vi "ConfigureSounds.vi"(11 "File":string="soundconfig.xml") -> (1 "Sound Cluster":T1={"Start"={"total number of samples/ch"=31680, "sound format"={"sample rate (S/s)"=11025.0, "number of channels"=1, "bits per sample"=16}, "data"=[{"t0"=timestamp(0 s since 1904-01-01), "dt"=9.070294784580499e-05, "Y"=array[31680 elements]}], "Volume"=100.0}, "Stop"={"total number of samples/ch"=27648, "sound format"={"sample rate (S/s)"=11025.0, "number of channels"=1, "bits per sample"=16}, "data"=[{"t0"=timestamp(0 s since 1904-01-01), "dt"=9.070294784580499e-05, "Y"=array[27648 elements]}], "Volume"=100.0}, "Uh-Oh"={"total number of samples/ch"=29952, "sound format"={"sample rate (S/s)"=11025.0, "number of channels"=1, "bits per sample"=16}, "data"=[{"t0"=timestamp(0 s since 1904-01-01), "dt"=9.070294784580499e-05, "Y"=array[29952 elements]}], "Volume"=88.46153846153847}, "PreMatch"={"total number of samples/ch"=225792, "sound format"={"sample rate (S/s)"=44100.0, "number of channels"=2, "bits per sample"=16}, "data"=[{"t0"=timestamp(0 s since 1904-01-01), "dt"=2.2675736961451248e-05, "Y"=array[225792 elements]}, {"t0"=timestamp(0 s since 1904-01-01), "dt"=2.2675736961451248e-05, "Y"=array[225792 elements]}], "Volume"=75.38461538461539}, "Hurry-Up"={"total number of samples/ch"=0, "sound format"={"sample rate (S/s)"=0.0, "number of channels"=0, "bits per sample"=0}, "data"=[], "Volume"=0.0}}, 3 "output cluster":T4)   [LabVIEW 2013]
uses:
  Sound Info.ctl
  <vilib>/sound2/lvsound2.llb/Sound Data Format.ctl
  <vilib>/Utility/sysdir.llb/System Directory Type.ctl
  <vilib>/sound2/lvsound2.llb/Sampling Mode.ctl
  <vilib>/Utility/xml.llb/Read From XML File(string).vi
  <vilib>/Utility/xml.llb/Write to XML File(string).vi
  <vilib>/sound2/lvsound2.llb/Sound Output Set Volume (Single).vi
  <vilib>/sound2/lvsound2.llb/Sound Output Write (DBL).vi
panel:
  in  "stop":bool
  in  "Sound To Play":T3(ring)
  in  "Tab Control":enum32{"Page 1", "Page 2"}(tab)
  in  "Cancel Button":bool
  in  "OK Button":bool
  in  "Test Hurry Up Sound":bool
  in  "Load Hurry Up Sound":bool
  in  "Hurry Up Sound Volume":dbl(slide)=88.46153846153847 scale=0.0..100.0
  in  "Hurry Up Sound":path=path "C:/ProgramData/FLL/sounds/TimeToRun.wav"
  in  "Test Pre-Match Sound":bool
  in  "Load Pre-Match Sound":bool
  in  "Pre-Match Coundown Sound Volume":dbl(slide)=88.46153846153847 scale=0.0..100.0
  in  "Pre-Match Countdown Sound":path=path "Z:/Code/LabVIEW/FLL 2.1/sounds/FOGHORN.wav"
  in  "Test Uh-Oh Sound":bool
  in  "Load Uh-Oh Sound":bool
  in  "Uh-Oh Sound Volume":dbl(slide)=88.46153846153847 scale=0.0..100.0
  in  "Uh-Oh Sound Path":path=path "Z:/Code/LabVIEW/FLL 2.1/sounds/FOGHORN.wav"
  in  "Test Stop Sound":bool
  in  "Load Stop Sound":bool
  in  "Stop Sound Volume":dbl(slide)=100.0 scale=0.0..100.0
  in  "Stop Sound Path":path=path "Z:/Code/LabVIEW/FLL 2.1/sounds/BUZZER.wav"
  in  "Test Start Sound":bool
  in  "Load Start Sound":bool
  in  "Start Sound Volume":dbl(slide)=100.0 scale=0.0..100.0
  in  "Start Sound Path":path=path "Z:/Code/LabVIEW/FLL 2.1/sounds/CHARGE.wav"
  in  "Master Volume":dbl(slide)=100.0 min=1.0 scale=0.0..100.0
  in  "Secondary (s)":dbl
  in  "Primary (s)":dbl=150.0
  in  "Pre-Primary (s)":dbl
  # "5"
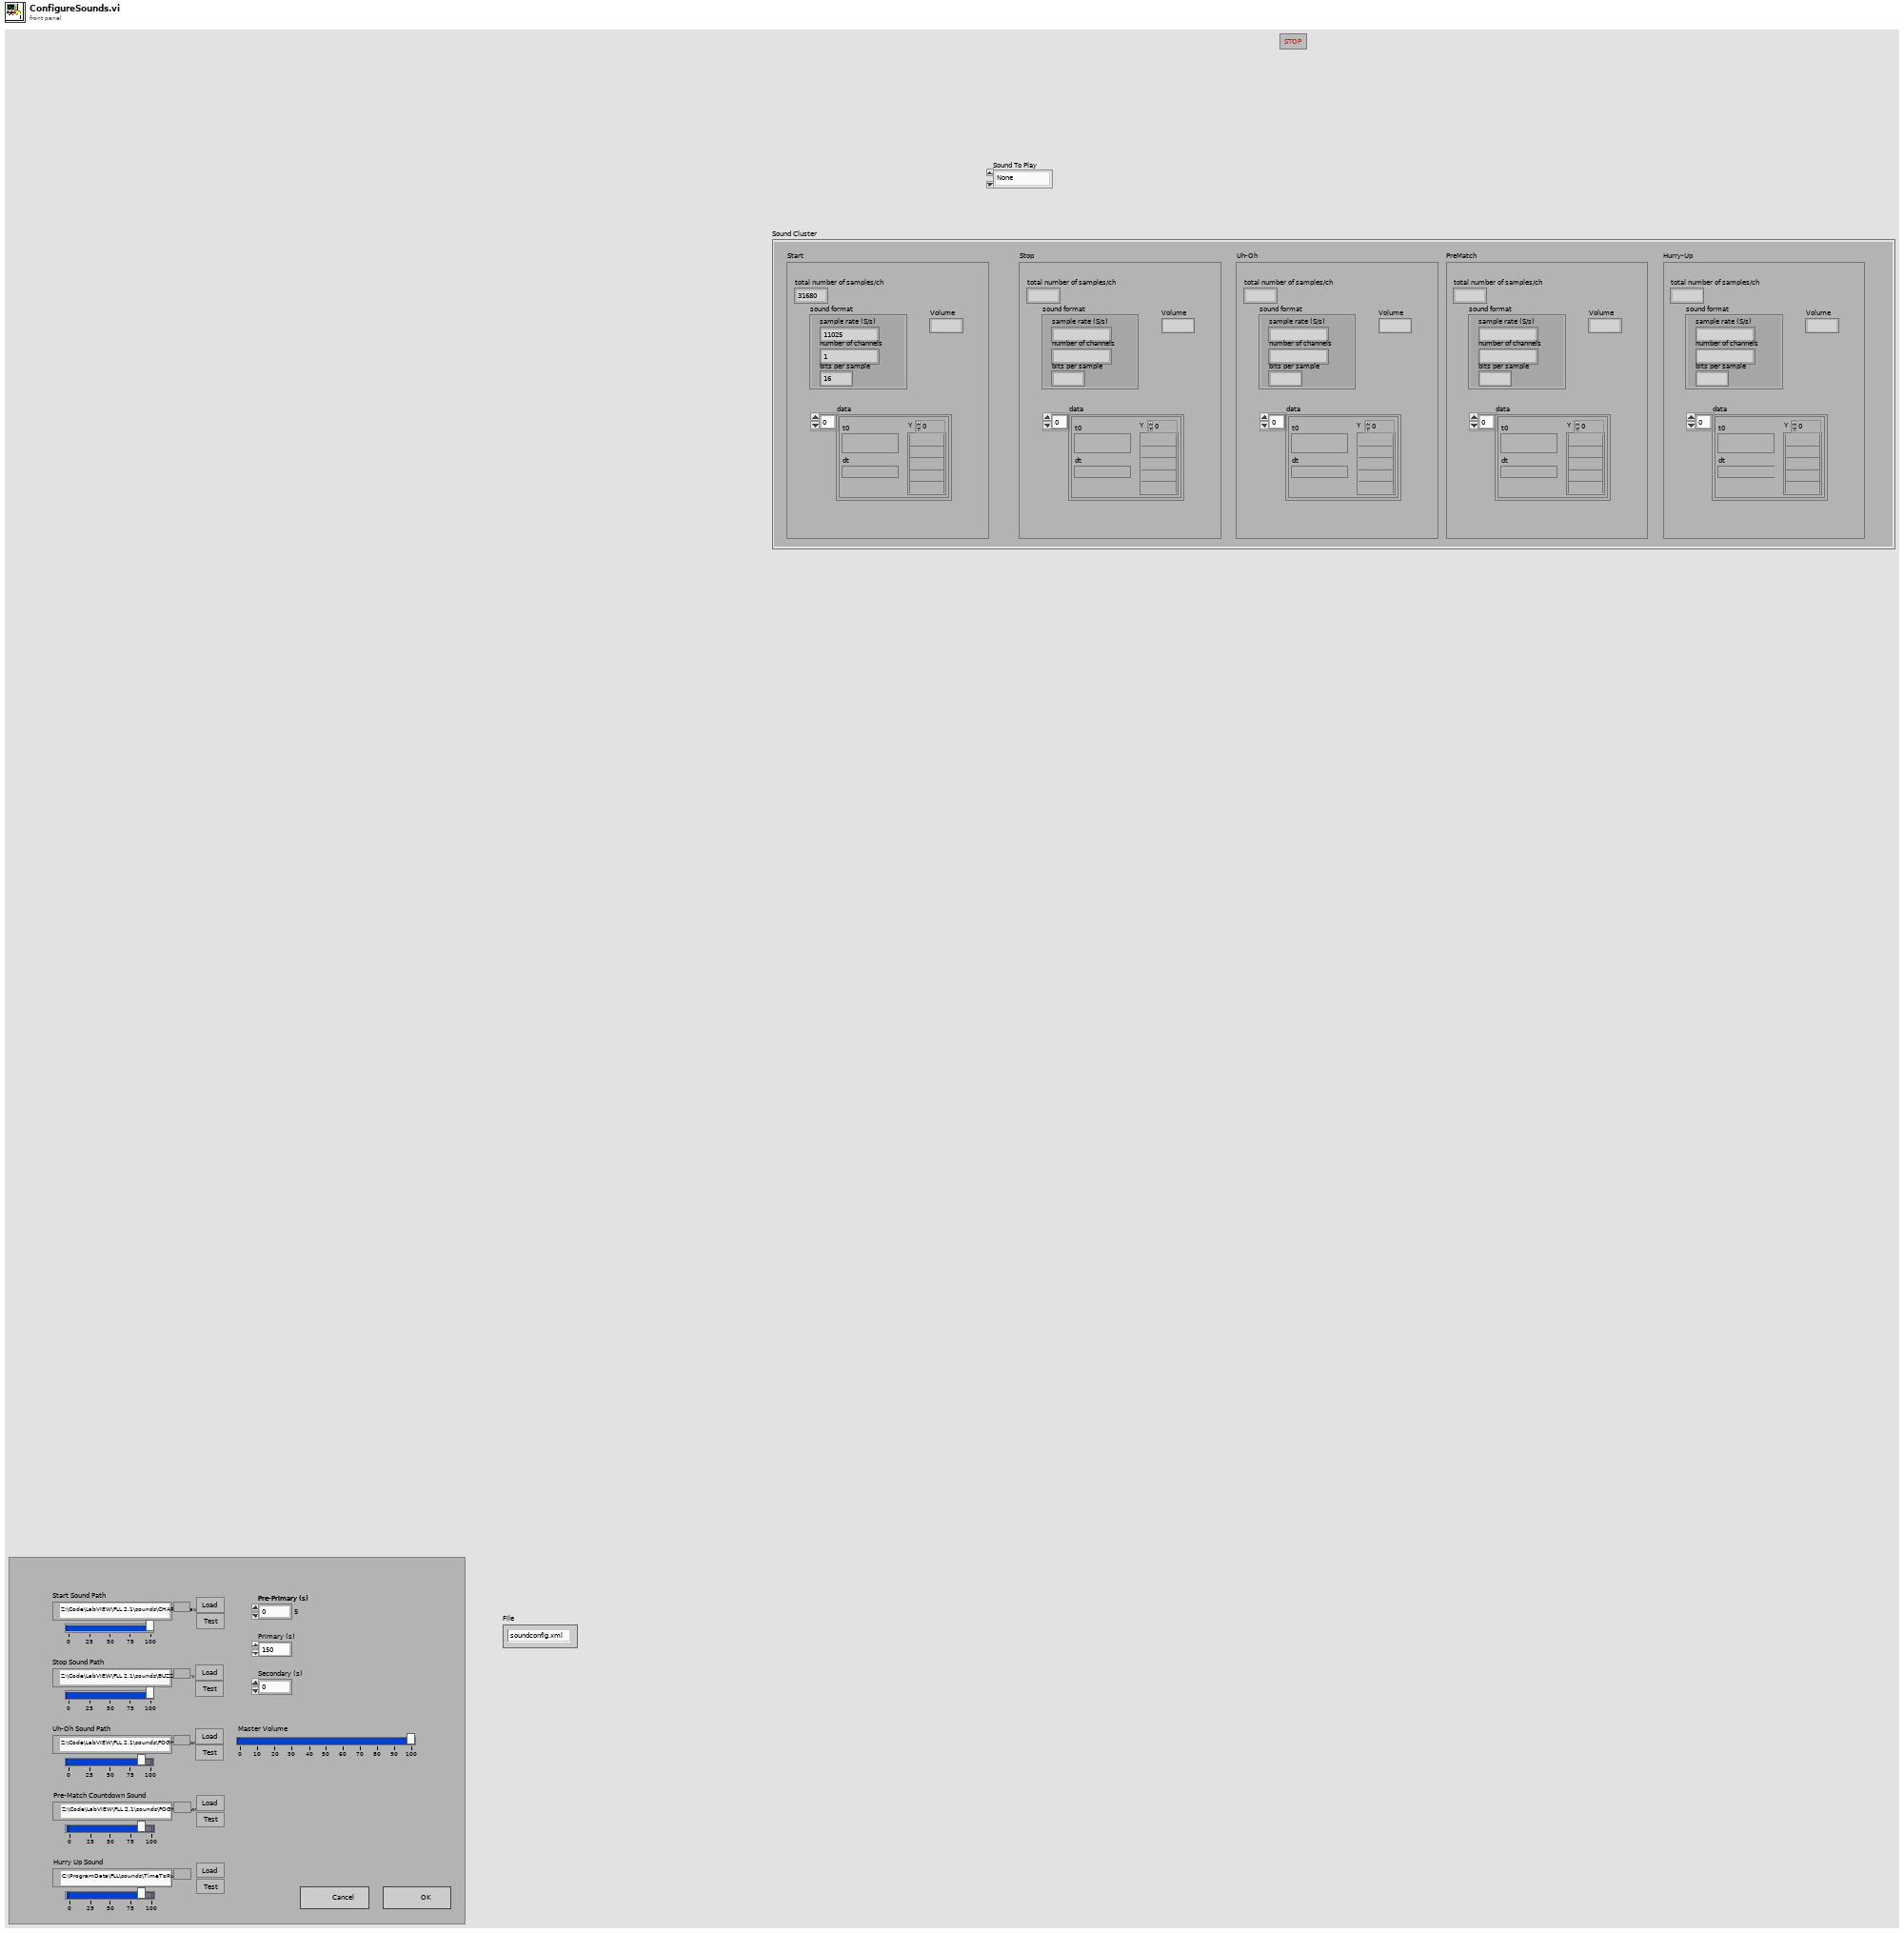
[diagram p1: front panel]
types:
  T1 = typedef "Sound Info.ctl" = cluster{"Start":cluster{"total number of samples/ch":u32, "sound format":T2, "data":waveform(dbl)[], "Volume":dbl}, "Stop":cluster{"total number of samples/ch":u32, "sound format":T2, "data":waveform(dbl)[], "Volume":dbl}, "Uh-Oh":cluster{"total number of samples/ch":u32, "sound format":T2, "data":waveform(dbl)[], "Volume":dbl}, "PreMatch":cluster{"total number of samples/ch":u32, "sound format":T2, "data":waveform(dbl)[], "Volume":dbl}, "Hurry-Up":cluster{"total number of samples/ch":u32, "sound format":T2, "data":waveform(dbl)[], "Volume":dbl}}
  T2 = typedef "Sound Data Format.ctl" = cluster{"sample rate (S/s)":dbl, "number of channels":i32, "bits per sample":i32}
  T3 = enum16{"None", "Start", "Stop", "Uh-Oh", "Prematch", "Hurry-Up"}
  T4 = cluster{"Master Volume":dbl, "Pre-Primary (s)":dbl, "Primary (s)":dbl, "Secondary (s)":dbl, "Start Sound Path":path, "Stop Sound Path":path, "Uh-Oh Sound Path":path, "Pre-Match Countdown Sound":path, "Hurry Up Sound":path, "Start Sound Volume":dbl, "Stop Sound Volume":dbl, "Uh-Oh Sound Volume":dbl, "Pre-Match Coundown Sound Volume":dbl, "Hurry Up Sound Volume":dbl}
  T5 = typedef "System Directory Type.ctl" = i32
  T6 = cluster{"total number of samples/ch":u32, "sound format":T2, "data":waveform(dbl)[], "Volume":dbl}
  T7 = typedef "Sampling Mode.ctl" = i32
  T8 = typedef "Sound Output Task ID.ctl" = u32
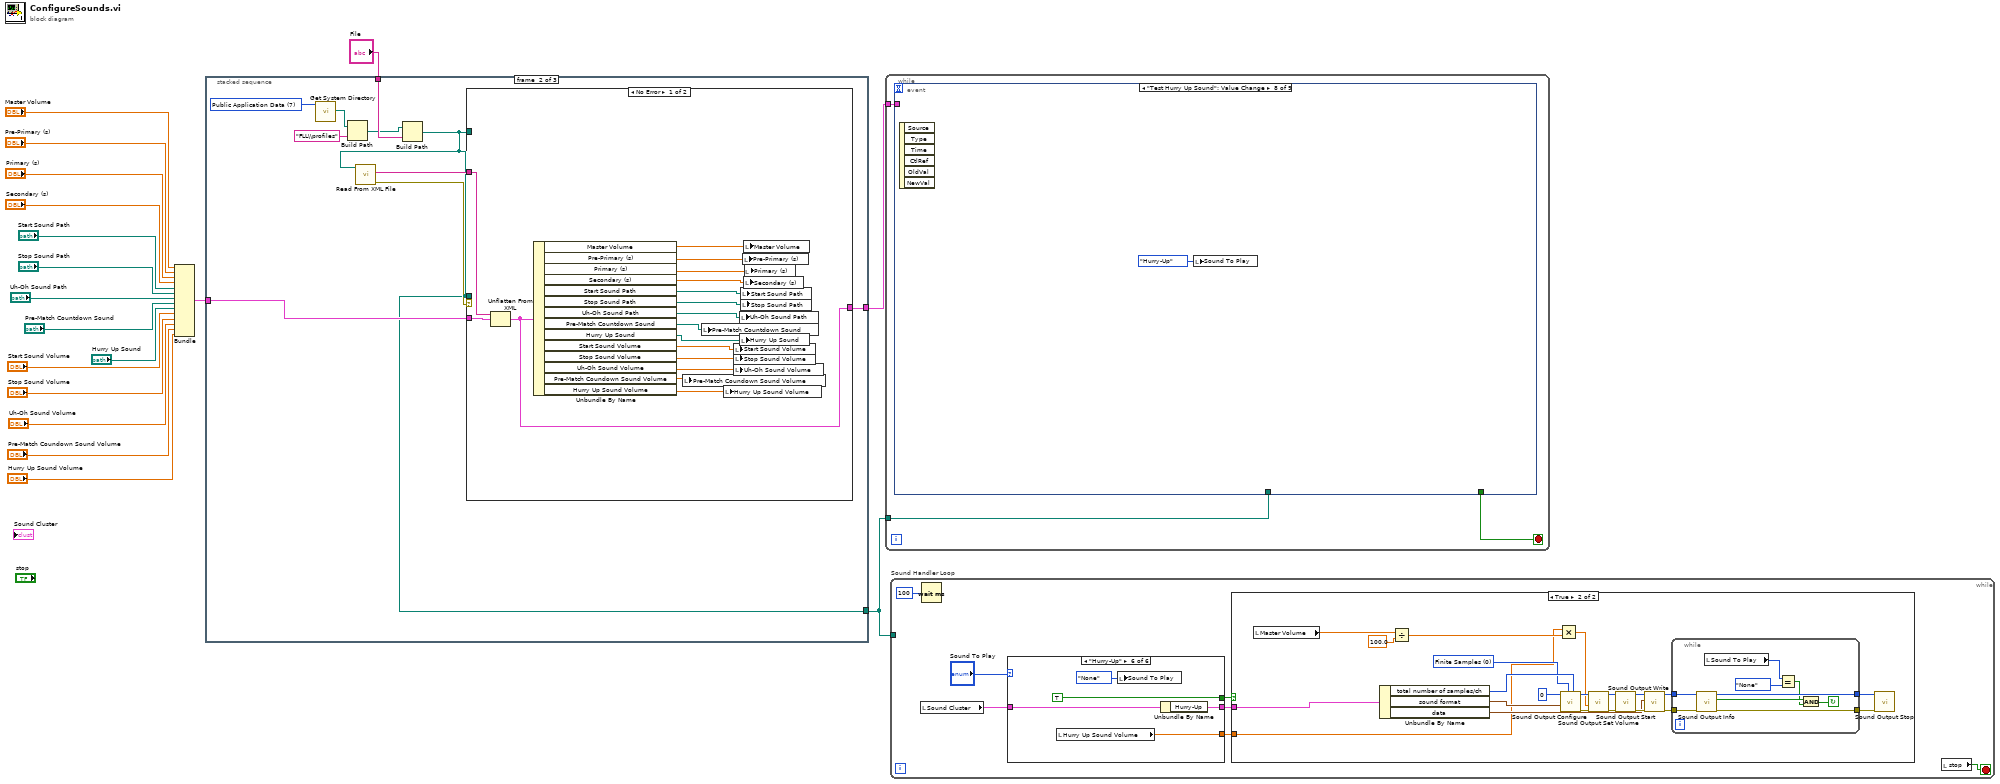
[diagram p0: block diagram]
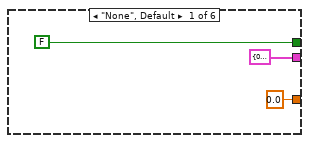
[diagram p3: hidden frame]
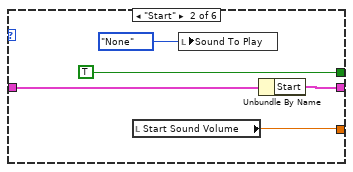
[diagram p4: hidden frame]
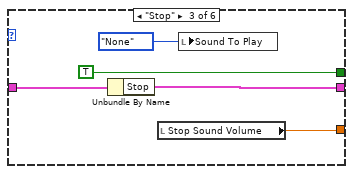
[diagram p5: hidden frame]
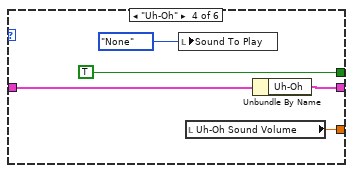
[diagram p6: hidden frame]
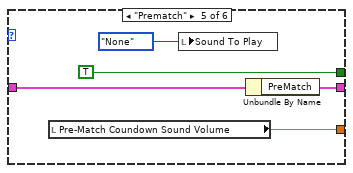
[diagram p7: hidden frame]
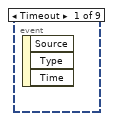
[diagram p8: hidden frame]
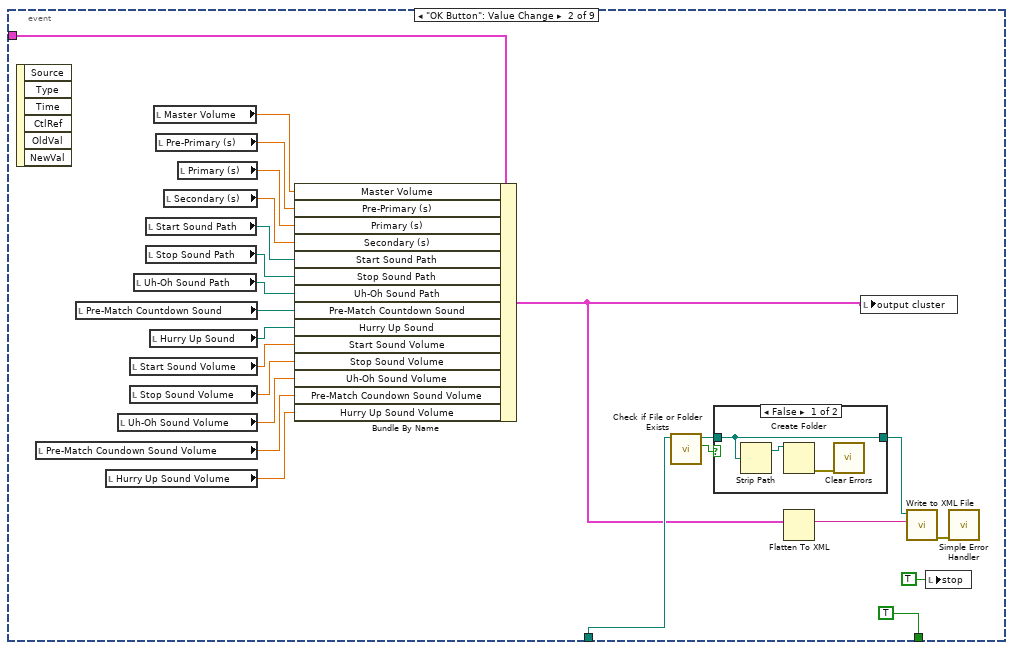
[diagram p9: hidden frame]
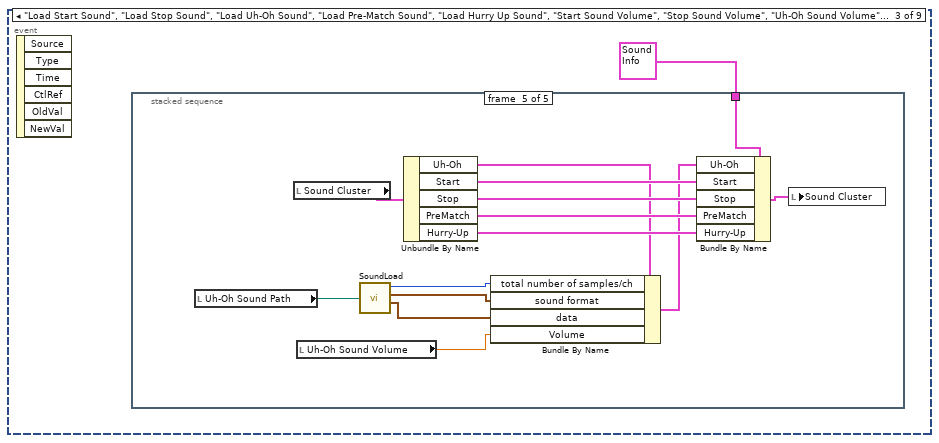
[diagram p11: hidden frame]
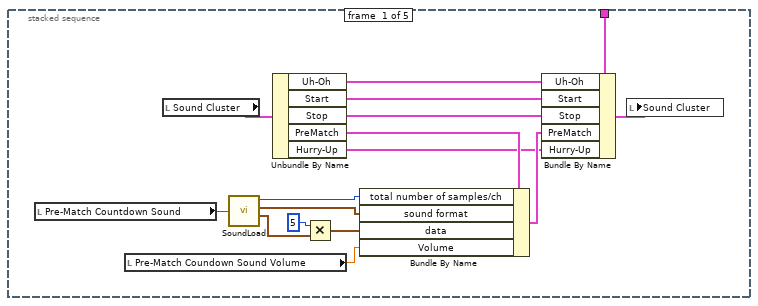
[diagram p12: hidden frame]
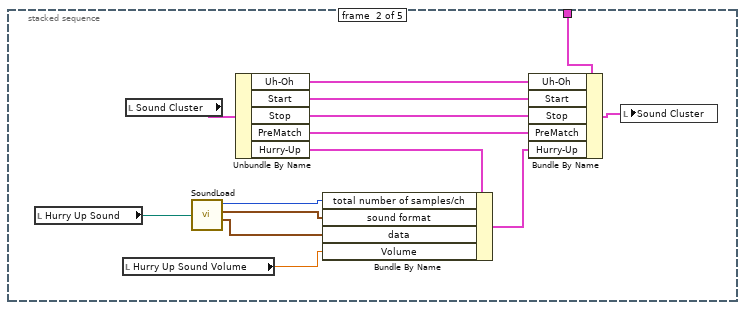
[diagram p13: hidden frame]
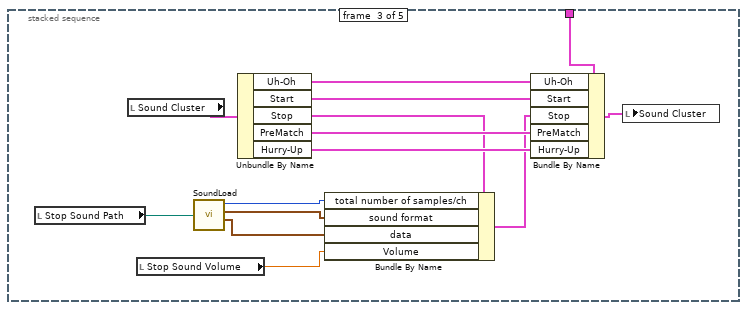
[diagram p14: hidden frame]
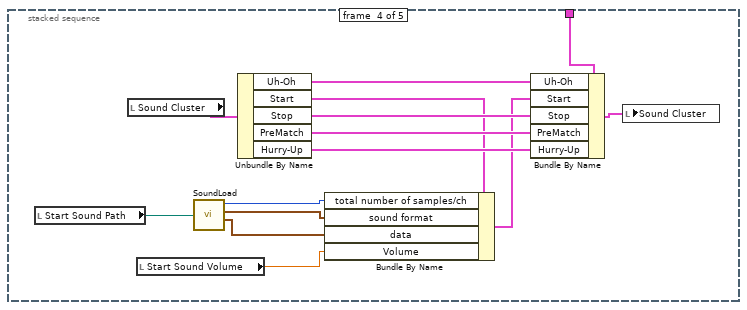
[diagram p15: hidden frame]
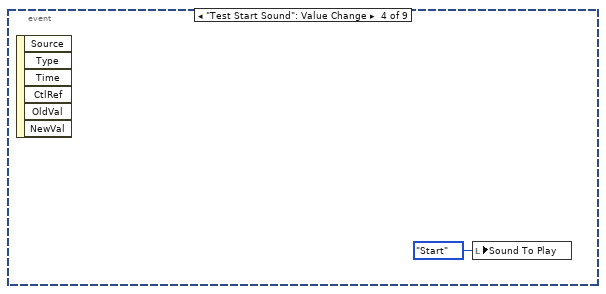
[diagram p16: hidden frame]
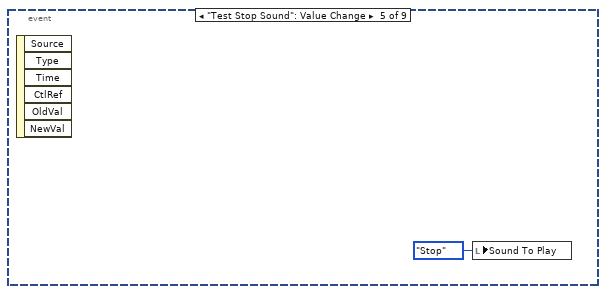
[diagram p17: hidden frame]
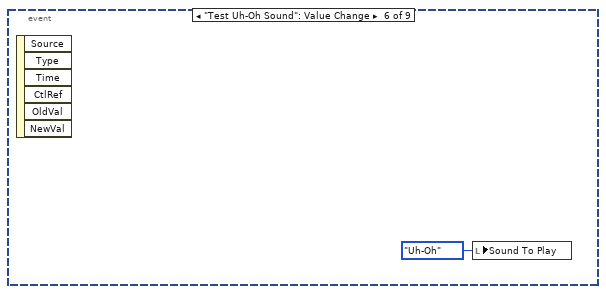
[diagram p18: hidden frame]
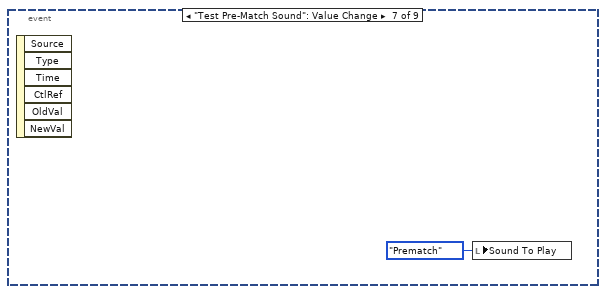
[diagram p19: hidden frame]
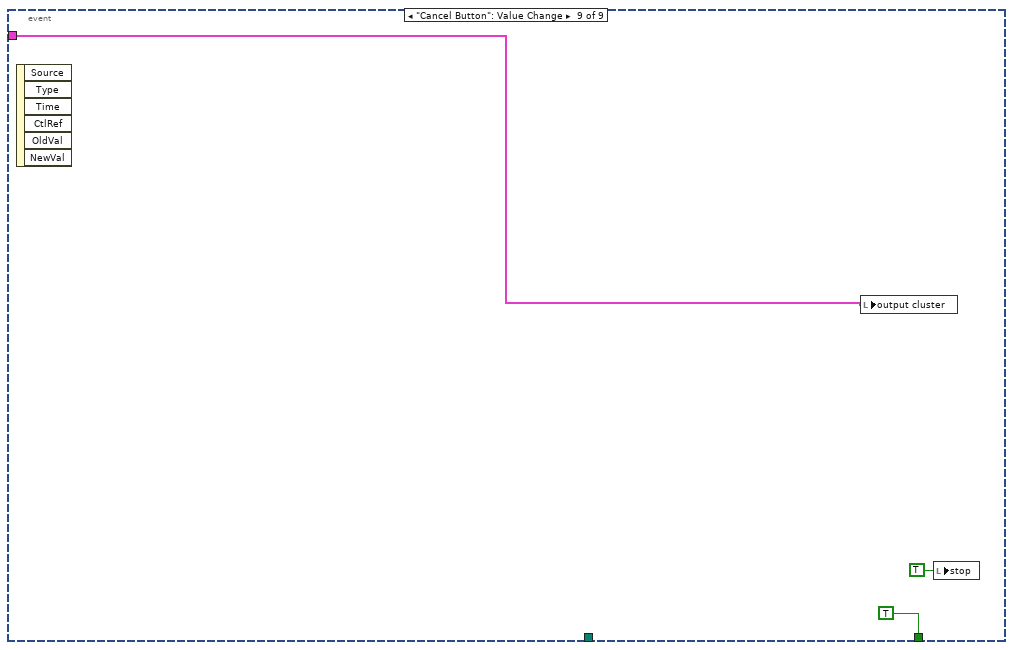
[diagram p20: hidden frame]
diagram:
  n1 = Bundle("Master Volume"="Master Volume", "Pre-Primary (s)"="Pre-Primary (s)", "Primary (s)"="Primary (s)", "Secondary (s)"="Secondary (s)", "Start Sound Path"="Start Sound Path", "Stop Sound Path"="Stop Sound Path", "Uh-Oh Sound Path"="Uh-Oh Sound Path", "Pre-Match Countdown Sound"="Pre-Match Countdown Sound", "Hurry Up Sound"="Hurry Up Sound", "Start Sound Volume"="Start Sound Volume", "Stop Sound Volume"="Stop Sound Volume", "Uh-Oh Sound Volume"="Uh-Oh Sound Volume", "Pre-Match Coundown Sound Volume"="Pre-Match Coundown Sound Volume", "Hurry Up Sound Volume"="Hurry Up Sound Volume") -> (w4:T4)  [unwired: 1 in]
  n2 = stacked-sequence {
    tunnel: w4 -> [_ w36 _]
    tunnel: [_ w31 _] -> w2
    tunnel: [_ w34 _] -> w3
    tunnel: "File" -> [_ w33 _]
    frame #0 {
      n3 = local write "stop"(FALSE ("stop")) -> ()
      n4 = control-ref of="Test Pre-Match Sound"() -> (w25:refnum<vi>)
      n5 = control-ref of="Test Hurry Up Sound"() -> (w26:refnum<vi>)
      n6 = control-ref of="Test Uh-Oh Sound"() -> (w24:refnum<vi>)
      n7 = control-ref of="Test Stop Sound"() -> (w23:refnum<vi>)
      n8 = control-ref of="Test Start Sound"() -> (w22:refnum<vi>)
      n9 = control-ref of="Cancel Button"() -> (w28:refnum<vi>)
      n10 = control-ref of="OK Button"() -> (w27:refnum<vi>)
      n11 = Build Array(w28, w27, w26, w25, w24, w23, w22) -> (w21:refnum<vi>[])
      n12 = for {
        tunnel: w21 -> [w30] mode=indexing
        n13 = property class="Bool (strict)"(reference=w30, "Value"=FALSE) -> ()  [unwired: 1 in, 2 out]
      }
      n14 = local write "Tab Control"(enum32{"Page 1", "Page 2"}."Page 1" ("Tab Control")) -> ()
    }
    frame #1 {
      w40 = T5 7 items=["User Home"=0, "User Desktop"=1, "User Documents"=2, "User Application Data"=3, "User Preferences"=4, "User Temporary"=5, "Public Documents"=6, "Public Application Data"=7, "Public Preferences"=8, "Public Cache"=13, "System Core Libraries"=9, "System Installed Libraries"=10, "Application Files"=11, "Boot Volume Root"=12] ("system directory type")
      n15 = call <vilib>:"Get System Directory.vi"("system directory type"=w40) -> ("system directory"=w39:path)  [unwired: 10 in]
      n16 = Build Path(base path=w39, name or relative path="FLL\\profiles") -> (appended path=w32:path)
      n17 = Build Path(base path=w32, name or relative path=w33) -> (appended path=w31:path)
      n18 = call-poly <vilib>:"Read From XML File.vi"("XML File Path"=w31) -> ("error out"=w37:errorcluster, "XML Elements"=w35:string)  [unwired: 8 in, 1 out]
      n19 = case shown="No Error" w37 {
        tunnel: w31 -> [_ _]
        tunnel: w36 -> [w57 w58]
        tunnel: w35 -> [w56 _]
        tunnel: w31 -> [_ w61]
        tunnel: [w41 w58] -> w34
        frame No Error {
          n20 = Unflatten From XML(xml string=w56, type=w57) -> (value=w41:T4)  [unwired: 1 in, 1 out]
          n21 = Unbundle By Name(w41) -> ("Master Volume"=w55:dbl, "Pre-Primary (s)"=w54:dbl, "Primary (s)"=w53:dbl, "Secondary (s)"=w52:dbl, "Start Sound Path"=w51:path, "Stop Sound Path"=w50:path, "Uh-Oh Sound Path"=w49:path, "Pre-Match Countdown Sound"=w48:path, "Hurry Up Sound"=w47:path, "Start Sound Volume"=w46:dbl, "Stop Sound Volume"=w45:dbl, "Uh-Oh Sound Volume"=w44:dbl, "Pre-Match Coundown Sound Volume"=w43:dbl, "Hurry Up Sound Volume"=w42:dbl)
          n22 = local write "Pre-Match Coundown Sound Volume"(w43) -> ()
          n23 = local write "Pre-Match Countdown Sound"(w48) -> ()
          n24 = local write "Hurry Up Sound Volume"(w42) -> ()
          n25 = local write "Start Sound Volume"(w46) -> ()
          n26 = local write "Stop Sound Volume"(w45) -> ()
          n27 = local write "Uh-Oh Sound Volume"(w44) -> ()
          n28 = local write "Uh-Oh Sound Path"(w49) -> ()
          n29 = local write "Hurry Up Sound"(w47) -> ()
          n30 = local write "Start Sound Path"(w51) -> ()
          n31 = local write "Stop Sound Path"(w50) -> ()
          n32 = local write "Pre-Primary (s)"(w54) -> ()
          n33 = local write "Master Volume"(w55) -> ()
          n34 = local write "Secondary (s)"(w52) -> ()
          n35 = local write "Primary (s)"(w53) -> ()
        }
        frame Error {
          n36 = Path To String(path=w61) -> (string=w60:string)
          n37 = call "Build Text"("configfile"=w60) -> ("Result"=w59:string)  [unwired: 13 in, 1 out]
          n38 = call "Display Message to User"("Message"=w59) -> ()  [unwired: 9 in, 2 out]
        }
      }
    }
    frame #2 {
      n39 = stacked-sequence {
        tunnel: T1 {"Start"={"total number of samples/ch"=0, "sound format"={"sample rate (S/s)"=0.0, "number of channels"=0, "bits per sample"=0}, "data"=[], "Volume"=0.0}, "Stop"={"total number of samples/ch"=0, "sound format"={"sample rate (S/s)"=0.0, "number of channels"=0, "bits per sample"=0}, "data"=[], "Volume"=0.0}, "Uh-Oh"={"total number of samples/ch"=0, "sound format"={"sample rate (S/s)"=0.0, "number of channels"=0, "bits per sample"=0}, "data"=[], "Volume"=0.0}, "PreMatch"={"total number of samples/ch"=0, "sound format"={"sample rate (S/s)"=0.0, "number of channels"=0, "bits per sample"=0}, "data"=[], "Volume"=0.0}, "Hurry-Up"={"total number of samples/ch"=0, "sound format"={"sample rate (S/s)"=0.0, "number of channels"=0, "bits per sample"=0}, "data"=[], "Volume"=0.0}} ("Sound Info") -> [w77 w91 w105 w119 w133]
        frame #0 {
          n40 = local read "Pre-Match Countdown Sound"() -> (w68:path)
          n41 = local read "Pre-Match Coundown Sound Volume"() -> (w67:dbl)
          n42 = local read "Sound Cluster"() -> (w78:T1)
          n43 = call "SoundLoad.vi"("Sound File"=w68) -> ("total number of samples/ch"=w71:u32, "sound format"=w72:T2, "data"=w65:waveform(dbl)[])  [unwired: 1 out]
          n44 = Unbundle By Name(w78) -> ("Uh-Oh"=w69:T6, "Start"=w76:T6, "Stop"=w75:T6, "PreMatch"=w74:T6, "Hurry-Up"=w63:T6)
          n45 = Multiply(x=5, y=w65) -> (x*y=w64:waveform(dbl)[])
          n46 = Bundle By Name(cluster=w74, "total number of samples/ch"=w71, "sound format"=w72, "data"=w64, "Volume"=w67) -> (w73:T6)
          n47 = Bundle By Name(cluster=w77, "Uh-Oh"=w69, "Start"=w76, "Stop"=w75, "PreMatch"=w73, "Hurry-Up"=w63) -> (w70:T1)
          n48 = local write "Sound Cluster"(w70) -> ()
        }
        frame #1 {
          n49 = local read "Hurry Up Sound"() -> (w84:path)
          n50 = local read "Hurry Up Sound Volume"() -> (w83:dbl)
          n51 = local read "Sound Cluster"() -> (w92:T1)
          n52 = call "SoundLoad.vi"("Sound File"=w84) -> ("total number of samples/ch"=w87:u32, "sound format"=w88:T2, "data"=w79:waveform(dbl)[])  [unwired: 1 out]
          n53 = Unbundle By Name(w92) -> ("Uh-Oh"=w85:T6, "Start"=w90:T6, "Stop"=w89:T6, "PreMatch"=w82:T6, "Hurry-Up"=w81:T6)
          n54 = Bundle By Name(cluster=w81, "total number of samples/ch"=w87, "sound format"=w88, "data"=w79, "Volume"=w83) -> (w80:T6)
          n55 = Bundle By Name(cluster=w91, "Uh-Oh"=w85, "Start"=w90, "Stop"=w89, "PreMatch"=w82, "Hurry-Up"=w80) -> (w86:T1)
          n56 = local write "Sound Cluster"(w86) -> ()
        }
        frame #2 {
          n57 = local read "Stop Sound Path"() -> (w99:path)
          n58 = local read "Sound Cluster"() -> (w106:T1)
          n59 = local read "Stop Sound Volume"() -> (w98:dbl)
          n60 = call "SoundLoad.vi"("Sound File"=w99) -> ("total number of samples/ch"=w102:u32, "sound format"=w103:T2, "data"=w93:waveform(dbl)[])  [unwired: 1 out]
          n61 = Unbundle By Name(w106) -> ("Uh-Oh"=w100:T6, "Start"=w104:T6, "Stop"=w95:T6, "PreMatch"=w97:T6, "Hurry-Up"=w96:T6)
          n62 = Bundle By Name(cluster=w95, "total number of samples/ch"=w102, "sound format"=w103, "data"=w93, "Volume"=w98) -> (w94:T6)
          n63 = Bundle By Name(cluster=w105, "Uh-Oh"=w100, "Start"=w104, "Stop"=w94, "PreMatch"=w97, "Hurry-Up"=w96) -> (w101:T1)
          n64 = local write "Sound Cluster"(w101) -> ()
        }
        frame #3 {
          n65 = local read "Start Sound Path"() -> (w114:path)
          n66 = local read "Sound Cluster"() -> (w120:T1)
          n67 = local read "Start Sound Volume"() -> (w113:dbl)
          n68 = call "SoundLoad.vi"("Sound File"=w114) -> ("total number of samples/ch"=w117:u32, "sound format"=w118:T2, "data"=w107:waveform(dbl)[])  [unwired: 1 out]
          n69 = Unbundle By Name(w120) -> ("Uh-Oh"=w115:T6, "Start"=w109:T6, "Stop"=w110:T6, "PreMatch"=w112:T6, "Hurry-Up"=w111:T6)
          n70 = Bundle By Name(cluster=w109, "total number of samples/ch"=w117, "sound format"=w118, "data"=w107, "Volume"=w113) -> (w108:T6)
          n71 = Bundle By Name(cluster=w119, "Uh-Oh"=w115, "Start"=w108, "Stop"=w110, "PreMatch"=w112, "Hurry-Up"=w111) -> (w116:T1)
          n72 = local write "Sound Cluster"(w116) -> ()
        }
        frame #4 {
          n73 = local read "Uh-Oh Sound Path"() -> (w129:path)
          n74 = local read "Sound Cluster"() -> (w134:T1)
          n75 = local read "Uh-Oh Sound Volume"() -> (w128:dbl)
          n76 = call "SoundLoad.vi"("Sound File"=w129) -> ("total number of samples/ch"=w131:u32, "sound format"=w132:T2, "data"=w124:waveform(dbl)[])  [unwired: 1 out]
          n77 = Unbundle By Name(w134) -> ("Uh-Oh"=w122:T6, "Start"=w123:T6, "Stop"=w125:T6, "PreMatch"=w127:T6, "Hurry-Up"=w126:T6)
          n78 = Bundle By Name(cluster=w122, "total number of samples/ch"=w131, "sound format"=w132, "data"=w124, "Volume"=w128) -> (w121:T6)
          n79 = Bundle By Name(cluster=w133, "Uh-Oh"=w121, "Start"=w123, "Stop"=w125, "PreMatch"=w127, "Hurry-Up"=w126) -> (w130:T1)
          n80 = local write "Sound Cluster"(w130) -> ()
        }
      }
    }
  }
  n81 = while {
    tunnel: w3 -> [w137]
    tunnel: w2 -> [w136]
    stop <- w135 stop-if-true
    n82 = event shown="[7] \"Test Hurry Up Sound\": Value Change" {
      selector: _ -> [_ _ _ _ _ _ _ _ _]
      dyn-events: _ -> [_ _ _ _ _ _ _ _ _]
      timeout: _ -> [_ _ _ _ _ _ _ _ _]
      tunnel: w137 -> [_ w161 _ _ _ _ _ _ w245]
      tunnel: w136 -> [_ w145 _ _ _ _ _ _ _]
      tunnel: [_ TRUE _ _ _ _ _ _ TRUE] -> w135
      event Timeout {
        n83 = event-data() -> ()  [unwired: 1 in, 3 out]
      }
      event "OK Button": Value Change {
        n84 = event-data() -> ()  [unwired: 1 in, 6 out]
        n85 = local read "Pre-Match Coundown Sound Volume"() -> (w148:dbl)
        n86 = local read "Pre-Match Countdown Sound"() -> (w153:path)
        n87 = local read "Hurry Up Sound Volume"() -> (w147:dbl)
        n88 = local read "Uh-Oh Sound Volume"() -> (w149:dbl)
        n89 = local read "Start Sound Volume"() -> (w151:dbl)
        n90 = local read "Stop Sound Volume"() -> (w150:dbl)
        n91 = local read "Uh-Oh Sound Path"() -> (w154:path)
        n92 = local read "Start Sound Path"() -> (w156:path)
        n93 = local read "Stop Sound Path"() -> (w155:path)
        n94 = local read "Hurry Up Sound"() -> (w152:path)
        n95 = local read "Master Volume"() -> (w160:dbl)
        n96 = local read "Pre-Primary (s)"() -> (w159:dbl)
        n97 = local read "Secondary (s)"() -> (w157:dbl)
        n98 = local read "Primary (s)"() -> (w158:dbl)
        n99 = Bundle By Name(cluster=w161, "Master Volume"=w160, "Pre-Primary (s)"=w159, "Primary (s)"=w158, "Secondary (s)"=w157, "Start Sound Path"=w156, "Stop Sound Path"=w155, "Uh-Oh Sound Path"=w154, "Pre-Match Countdown Sound"=w153, "Hurry Up Sound"=w152, "Start Sound Volume"=w151, "Stop Sound Volume"=w150, "Uh-Oh Sound Volume"=w149, "Pre-Match Coundown Sound Volume"=w148, "Hurry Up Sound Volume"=w147) -> (w139:T4)
        n100 = call <vilib>:"Check if File or Folder Exists.vi"("path"=w145) -> ("file or folder exists?"=w144:bool, "dup path"=w143:path)  [unwired: 8 in, 1 out]
        n101 = case shown="False" w144 {
          tunnel: w143 -> [w163 w165]
          tunnel: [w163 w165] -> w142
          frame False {
            n102 = Strip Path(path=w163) -> (stripped path=w164:path)  [unwired: 1 out]
            n103 = Create Folder(path (use dialog)=w164) -> (error out=w162:errorcluster)  [unwired: 2 in, 2 out]
            n104 = call <vilib>:"Clear Errors.vi"("error in (no error)"=w162) -> ()  [unwired: 6 in, 1 out]
          }
          frame True {
          }
        }
        n105 = Flatten To XML(anything=w139) -> (xml string=w146:string)
        n106 = local write "output cluster"(w139) -> ()
        n107 = call-poly <vilib>:"Write to XML File.vi"("XML Input"=w146, "XML File Path"=w142) -> ("error out"=w141:errorcluster)  [unwired: 7 in, 2 out]
        n108 = local write "stop"(TRUE ("stop")) -> ()
        n109 = call <vilib>:"Simple Error Handler.vi"("error in (no error)"=w141) -> ()  [unwired: 4 in, 5 out]
      }
      event "Load Start Sound", "Load Stop Sound", "Load Uh-Oh Sound", "Load Pre-Match Sound", "Load Hurry Up Sound", "Start Sound Volume", "Stop Sound Volume", "Uh-Oh Sound Volume", "Pre-Match Coundown Sound Volume", "Hurry Up Sound Volume": Value Change {
        n110 = event-data() -> ()  [unwired: 1 in, 6 out]
        n111 = stacked-sequence {
          tunnel: T1 {"Start"={"total number of samples/ch"=0, "sound format"={"sample rate (S/s)"=0.0, "number of channels"=0, "bits per sample"=0}, "data"=[], "Volume"=0.0}, "Stop"={"total number of samples/ch"=0, "sound format"={"sample rate (S/s)"=0.0, "number of channels"=0, "bits per sample"=0}, "data"=[], "Volume"=0.0}, "Uh-Oh"={"total number of samples/ch"=0, "sound format"={"sample rate (S/s)"=0.0, "number of channels"=0, "bits per sample"=0}, "data"=[], "Volume"=0.0}, "PreMatch"={"total number of samples/ch"=0, "sound format"={"sample rate (S/s)"=0.0, "number of channels"=0, "bits per sample"=0}, "data"=[], "Volume"=0.0}, "Hurry-Up"={"total number of samples/ch"=0, "sound format"={"sample rate (S/s)"=0.0, "number of channels"=0, "bits per sample"=0}, "data"=[], "Volume"=0.0}} ("Sound Info") -> [w181 w195 w209 w223 w237]
          frame #0 {
            n112 = local read "Pre-Match Countdown Sound"() -> (w172:path)
            n113 = local read "Pre-Match Coundown Sound Volume"() -> (w171:dbl)
            n114 = local read "Sound Cluster"() -> (w182:T1)
            n115 = call "SoundLoad.vi"("Sound File"=w172) -> ("total number of samples/ch"=w175:u32, "sound format"=w176:T2, "data"=w169:waveform(dbl)[])  [unwired: 1 out]
            n116 = Unbundle By Name(w182) -> ("Uh-Oh"=w173:T6, "Start"=w180:T6, "Stop"=w179:T6, "PreMatch"=w178:T6, "Hurry-Up"=w167:T6)
            n117 = Multiply(x=5, y=w169) -> (x*y=w168:waveform(dbl)[])
            n118 = Bundle By Name(cluster=w178, "total number of samples/ch"=w175, "sound format"=w176, "data"=w168, "Volume"=w171) -> (w177:T6)
            n119 = Bundle By Name(cluster=w181, "Uh-Oh"=w173, "Start"=w180, "Stop"=w179, "PreMatch"=w177, "Hurry-Up"=w167) -> (w174:T1)
            n120 = local write "Sound Cluster"(w174) -> ()
          }
          frame #1 {
            n121 = local read "Hurry Up Sound"() -> (w188:path)
            n122 = local read "Hurry Up Sound Volume"() -> (w187:dbl)
            n123 = local read "Sound Cluster"() -> (w196:T1)
            n124 = call "SoundLoad.vi"("Sound File"=w188) -> ("total number of samples/ch"=w191:u32, "sound format"=w192:T2, "data"=w183:waveform(dbl)[])  [unwired: 1 out]
            n125 = Unbundle By Name(w196) -> ("Uh-Oh"=w189:T6, "Start"=w194:T6, "Stop"=w193:T6, "PreMatch"=w186:T6, "Hurry-Up"=w185:T6)
            n126 = Bundle By Name(cluster=w185, "total number of samples/ch"=w191, "sound format"=w192, "data"=w183, "Volume"=w187) -> (w184:T6)
            n127 = Bundle By Name(cluster=w195, "Uh-Oh"=w189, "Start"=w194, "Stop"=w193, "PreMatch"=w186, "Hurry-Up"=w184) -> (w190:T1)
            n128 = local write "Sound Cluster"(w190) -> ()
          }
          frame #2 {
            n129 = local read "Stop Sound Path"() -> (w203:path)
            n130 = local read "Sound Cluster"() -> (w210:T1)
            n131 = local read "Stop Sound Volume"() -> (w202:dbl)
            n132 = call "SoundLoad.vi"("Sound File"=w203) -> ("total number of samples/ch"=w206:u32, "sound format"=w207:T2, "data"=w197:waveform(dbl)[])  [unwired: 1 out]
            n133 = Unbundle By Name(w210) -> ("Uh-Oh"=w204:T6, "Start"=w208:T6, "Stop"=w199:T6, "PreMatch"=w201:T6, "Hurry-Up"=w200:T6)
            n134 = Bundle By Name(cluster=w199, "total number of samples/ch"=w206, "sound format"=w207, "data"=w197, "Volume"=w202) -> (w198:T6)
            n135 = Bundle By Name(cluster=w209, "Uh-Oh"=w204, "Start"=w208, "Stop"=w198, "PreMatch"=w201, "Hurry-Up"=w200) -> (w205:T1)
            n136 = local write "Sound Cluster"(w205) -> ()
          }
          frame #3 {
            n137 = local read "Start Sound Path"() -> (w218:path)
            n138 = local read "Sound Cluster"() -> (w224:T1)
            n139 = local read "Start Sound Volume"() -> (w217:dbl)
            n140 = call "SoundLoad.vi"("Sound File"=w218) -> ("total number of samples/ch"=w221:u32, "sound format"=w222:T2, "data"=w211:waveform(dbl)[])  [unwired: 1 out]
            n141 = Unbundle By Name(w224) -> ("Uh-Oh"=w219:T6, "Start"=w213:T6, "Stop"=w214:T6, "PreMatch"=w216:T6, "Hurry-Up"=w215:T6)
            n142 = Bundle By Name(cluster=w213, "total number of samples/ch"=w221, "sound format"=w222, "data"=w211, "Volume"=w217) -> (w212:T6)
            n143 = Bundle By Name(cluster=w223, "Uh-Oh"=w219, "Start"=w212, "Stop"=w214, "PreMatch"=w216, "Hurry-Up"=w215) -> (w220:T1)
            n144 = local write "Sound Cluster"(w220) -> ()
          }
          frame #4 {
            n145 = local read "Uh-Oh Sound Path"() -> (w233:path)
            n146 = local read "Sound Cluster"() -> (w238:T1)
            n147 = local read "Uh-Oh Sound Volume"() -> (w232:dbl)
            n148 = call "SoundLoad.vi"("Sound File"=w233) -> ("total number of samples/ch"=w235:u32, "sound format"=w236:T2, "data"=w228:waveform(dbl)[])  [unwired: 1 out]
            n149 = Unbundle By Name(w238) -> ("Uh-Oh"=w226:T6, "Start"=w227:T6, "Stop"=w229:T6, "PreMatch"=w231:T6, "Hurry-Up"=w230:T6)
            n150 = Bundle By Name(cluster=w226, "total number of samples/ch"=w235, "sound format"=w236, "data"=w228, "Volume"=w232) -> (w225:T6)
            n151 = Bundle By Name(cluster=w237, "Uh-Oh"=w225, "Start"=w227, "Stop"=w229, "PreMatch"=w231, "Hurry-Up"=w230) -> (w234:T1)
            n152 = local write "Sound Cluster"(w234) -> ()
          }
        }
      }
      event "Test Start Sound": Value Change {
        n153 = event-data() -> ()  [unwired: 1 in, 6 out]
        n154 = local write "Sound To Play"(T3."Start" ("Sound To Play")) -> ()
      }
      event "Test Stop Sound": Value Change {
        n155 = event-data() -> ()  [unwired: 1 in, 6 out]
        n156 = local write "Sound To Play"(T3."Stop" ("Sound To Play")) -> ()
      }
      event "Test Uh-Oh Sound": Value Change {
        n157 = event-data() -> ()  [unwired: 1 in, 6 out]
        n158 = local write "Sound To Play"(T3."Uh-Oh" ("Sound To Play")) -> ()
      }
      event "Test Pre-Match Sound": Value Change {
        n159 = event-data() -> ()  [unwired: 1 in, 6 out]
        n160 = local write "Sound To Play"(T3."Prematch" ("Sound To Play")) -> ()
      }
      event "Test Hurry Up Sound": Value Change {
        n161 = event-data() -> ()  [unwired: 1 in, 6 out]
        n162 = local write "Sound To Play"(T3."Hurry-Up" ("Sound To Play")) -> ()
      }
      event "Cancel Button": Value Change {
        n163 = event-data() -> ()  [unwired: 1 in, 6 out]
        n164 = local write "output cluster"(w245) -> ()
        n165 = local write "stop"(TRUE ("stop")) -> ()
      }
    }
  }
  n166 = while "Sound Handler Loop" {
    tunnel: w2 -> [_]
    stop <- w249 stop-if-true
    n167 = local read "Sound Cluster"() -> (w252:T1)
    n168 = Wait (ms)(milliseconds to wait=u32 100) -> ()  [unwired: 1 out]
    n169 = case shown="\"Hurry-Up\"" "Sound To Play" {
      tunnel: w252 -> [_ w291 w296 w301 w306 w311]
      tunnel: [T6 {"total number of samples/ch"=0, "sound format"={"sample rate (S/s)"=0.0, "number of channels"=0, "bits per sample"=0}, "data"=[], "Volume"=0.0} ("Uh-Oh") w290 w295 w299 w304 w310] -> w251
      tunnel: [FALSE TRUE TRUE TRUE TRUE TRUE] -> w250
      tunnel: [0.0 ("Pre-Match Coundown Sound Volume") w287 w292 w297 w302 w308] -> w247
      frame "None", Default {
      }
      frame "Start" {
        n170 = local read "Start Sound Volume"() -> (w287:dbl)
        n171 = local write "Sound To Play"(enum16{"None", "Start", "Stop", "Uh-Oh"}."None" ("Sound To Play")) -> ()
        n172 = Unbundle By Name(w291) -> ("Start"=w290:T6)
      }
      frame "Stop" {
        n173 = Unbundle By Name(w296) -> ("Stop"=w295:T6)
        n174 = local read "Stop Sound Volume"() -> (w292:dbl)
        n175 = local write "Sound To Play"(enum16{"None", "Start", "Stop", "Uh-Oh"}."None" ("Sound To Play")) -> ()
      }
      frame "Uh-Oh" {
        n176 = local write "Sound To Play"(enum16{"None", "Start", "Stop", "Uh-Oh"}."None" ("Sound To Play")) -> ()
        n177 = local read "Uh-Oh Sound Volume"() -> (w297:dbl)
        n178 = Unbundle By Name(w301) -> ("Uh-Oh"=w299:T6)
      }
      frame "Prematch" {
        n179 = local read "Pre-Match Coundown Sound Volume"() -> (w302:dbl)
        n180 = local write "Sound To Play"(enum16{"None", "Start", "Stop", "Uh-Oh"}."None" ("Sound To Play")) -> ()
        n181 = Unbundle By Name(w306) -> ("PreMatch"=w304:T6)
      }
      frame "Hurry-Up" {
        n182 = local read "Hurry Up Sound Volume"() -> (w308:dbl)
        n183 = local write "Sound To Play"(T3."None" ("Sound To Play")) -> ()
        n184 = Unbundle By Name(w311) -> ("Hurry-Up"=w310:T6)
      }
    }
    n185 = case shown="True" w250 {
      tunnel: w251 -> [_ w274]
      tunnel: w247 -> [_ w255]
      frame False {
      }
      frame True {
        w272 = T7 0 items=["Finite Samples", "Continuous Samples"] ("sample mode")
        n186 = local read "Master Volume"() -> (w254:dbl)
        n187 = Unbundle By Name(w274) -> ("total number of samples/ch"=w273:u32, "sound format"=w271:T2, "data"=w264:waveform(dbl)[])
        n188 = Divide(x=w254, y=100.0) -> (x/y=w258:dbl)
        n189 = Multiply(x=w255, y=w258) -> (x*y=w257:dbl)
        n190 = call <vilib>:"Sound Output Configure.vi"("number of samples/ch"=w273, "sample mode"=w272, "sound format"=w271, "device ID"=u32 0) -> ("error out"=w269:errorcluster, "task ID"=w270:T8)  [unwired: 6 in]
        n191 = call-poly <vilib>:"Sound Output Set Volume.vi"("error in (no error)"=w269, "volume"=w257, "task ID"=w270) -> ("error out"=w267:errorcluster, "task ID out"=w268:T8)  [unwired: 7 in]
        n192 = call <vilib>:"Sound Output Start.vi"("error in (no error)"=w267, "task ID"=w268) -> ("error out"=w265:errorcluster, "task ID out"=w266:T8)  [unwired: 8 in]
        n193 = call-poly <vilib>:"Sound Output Write.vi"("error in (no error)"=w265, "data"=w264, "task ID"=w266) -> ("error out"=w262:errorcluster, "task ID out"=w263:T8)  [unwired: 7 in]
        n194 = while {
          tunnel: w263 -> [w283]
          tunnel: w262 -> [w282]
          tunnel: [w281] -> w261
          tunnel: [w280] -> w260
          stop <- w275 continue-if-true
          n195 = call <vilib>:"Sound Output Info.vi"("error in (no error)"=w282, "task ID"=w283) -> ("error out"=w280:errorcluster, "is playing?"=w279:bool, "task ID out"=w281:T8)  [unwired: 6 in, 1 out]
          n196 = local read "Sound To Play"() -> (w277:T3)
          n197 = Equal?(x=w277, y=enum16{"None", "Start", "Stop", "Uh-Oh"}."None") -> (x = y?=w278:bool)
          n198 = And(x=w279, y=w278) -> (x .and. y?=w275:bool)
        }
        n199 = call <vilib>:"Sound Output Stop.vi"("error in (no error)"=w260, "task ID"=w261) -> ()  [unwired: 8 in, 2 out]
      }
    }
    n200 = local read "stop"() -> (w249:bool)
  }
